vi "REWORK_TCP_check_for_error.vi"(8 "PLC_TCP_loop_state_in":T1, 11 "error_in":errorcluster) -> (0 "PLC_TCP_loop_state_out":T1, 3 "error_out":errorcluster)   [LabVIEW 2019]
uses:
  REWORK_TCP_sequence_state.ctl
  FGV/connection_reference/FGV_REWORK_connection_reference.ctl
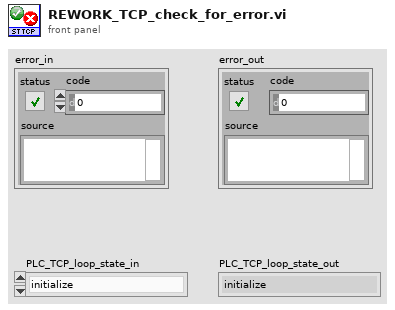
[diagram p1: front panel]
types:
  T1 = typedef "REWORK_TCP_sequence_state.ctl" = enum16{"initialize", "wait_for_connection", "handle_message", "error", "stop"}
  T2 = typedef "FGV_REWORK_connection_reference.ctl" = enum16{"initialize", "set_listener_ID", "set_connection_ID", "get", "KILL_ALL_CONNECTIONS", "killed?"}
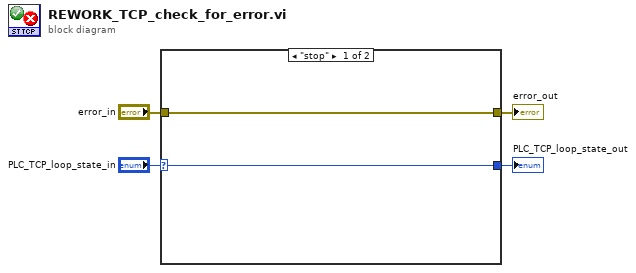
[diagram p0: block diagram]
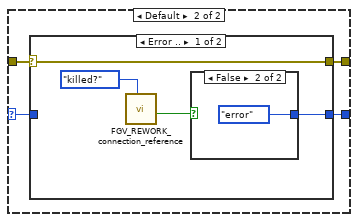
[diagram p2: hidden frame]
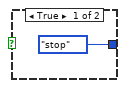
[diagram p3: hidden frame]
diagram:
  n1 = case shown="\"stop\"" "PLC_TCP_loop_state_in" {
    selector: "PLC_TCP_loop_state_in" -> [w5 w8]
    tunnel: [w6 w10] -> w4
    tunnel: [w5 w9] -> w3
    tunnel: "error_in" -> [w6 w7]
    frame "stop" {
    }
    frame Default {
      n2 = case shown="Error .." w7 {
        selector: w7 -> [w13 w17]
        tunnel: [w14 w18] -> w9
        tunnel: w8 -> [_ w18]
        tunnel: [w13 w17] -> w10
        frame Error {
          n3 = call "FGV_REWORK_connection_reference.vi"("options"=FGV_REWORK_connection_reference."killed?") -> ("killed?"=w11:bool)  [unwired: 7 in, 3 out]
          n4 = case shown="False" w11 {
            tunnel: [REWORK_TCP_sequence_state."stop" ("PLC_TCP_1_loop_states") REWORK_TCP_sequence_state."error" ("PLC_TCP_1_loop_states")] -> w14
            frame True {
            }
            frame False {
            }
          }
        }
        frame No Error {
        }
      }
    }
  }
  "error_out" <- w4
  "PLC_TCP_loop_state_out" <- w3
